vi "Find Parse State Queue from While Loop.vi"(8 "error in (no error)":errorcluster, 11 "WhileLoop in":refnum<vi>) -> (0 "error out":errorcluster, 1 "CaseStructure":refnum<vi>, 2 "Parse State Queue":refnum<vi>, 3 "WhileLoop out":refnum<vi>)   [LabVIEW 2020, in "CSM-Helper.lvclass"]
uses:
  CSM-Helper.lvclass
  CSM-Helper.lvclass/CSM-Helper.ctl
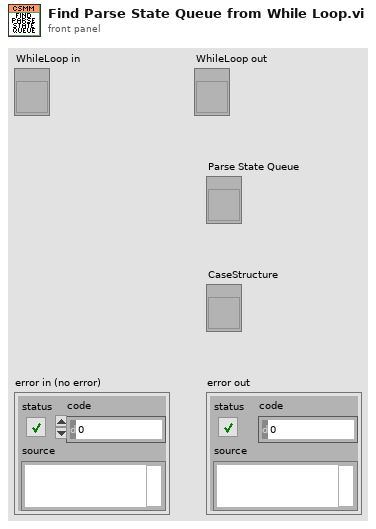
[diagram p1: front panel]
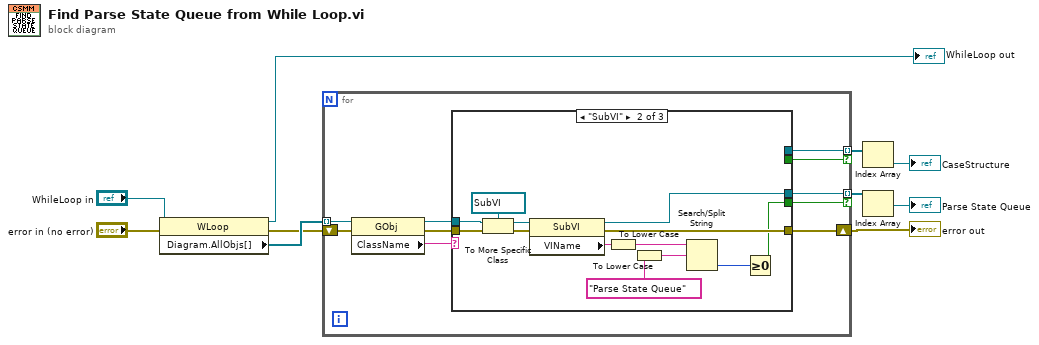
[diagram p0: block diagram]
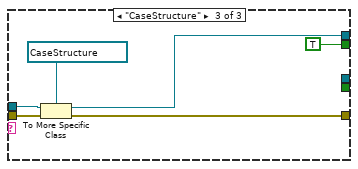
[diagram p3: hidden frame]
diagram:
  n1 = property on="Property Node" class="WLoop"(reference="WhileLoop in", error in="error in (no error)") -> (reference out=→"WhileLoop out":refnum<vi>, error out=w7:errorcluster, "Diagram.AllObjs[]"=w10:refnum<vi>[])
  n2 = for {
    tunnel: w10 -> [w20] mode=indexing
    shift-right: [w15] -> w6
    shift-left: w7 -> [w16]
    tunnel: [w14] -> w3 mode=indexing if=w11
    tunnel: [w13] -> w5 mode=indexing if=w12
    n3 = property class="GObj"(reference=w20, error in=w16) -> (reference out=w18:refnum<vi>, error out=w17:errorcluster, "ClassName"=w19:string)
    n4 = case shown="\"SubVI\"" w19 {
      tunnel: w18 -> [_ w33 w39]
      tunnel: w17 -> [w21 w32 w38]
      tunnel: [w21 w27 w37] -> w15
      tunnel: [_ w26 _] -> w14
      tunnel: [_ _ w36] -> w13
      tunnel: [_ _ TRUE] -> w12
      tunnel: [_ w22 _] -> w11
      frame Default {
      }
      frame "SubVI" {
        n5 = To More Specific Class(target class=refnum<vi> refnum ("SubVI Refnum"), reference=w33, error in=w32) -> (specific class reference=w31:refnum<vi>, error out=w30:errorcluster)
        n6 = property class="SubVI"(reference=w31, error in=w30) -> (reference out=w26:refnum<vi>, error out=w27:errorcluster, "VIName"=w29:string)
        n7 = To Lower Case(string=w29) -> (all lower case string=w24:string)
        n8 = To Lower Case(string="Parse State Queue" ("VI Name")) -> (all lower case string=w25:string)
        n9 = Search/Split String(string=w24, search string/char (-)=w25) -> (offset of match=w23:i32)  [unwired: 1 in, 2 out]
        n10 = Greater Or Equal To 0?(x=w23) -> (x >= 0?=w22:bool)
      }
      frame "CaseStructure" {
        n11 = To More Specific Class(target class=refnum<vi> refnum ("CaseSel Refnum"), reference=w39, error in=w38) -> (specific class reference=w36:refnum<vi>, error out=w37:errorcluster)
      }
    }
  }
  "error out" <- w6
  n12 = Index Array(array=w5) -> (element=→"CaseStructure":refnum<vi>)  [unwired: 1 in]
  n13 = Index Array(array=w3) -> (element=→"Parse State Queue":refnum<vi>)  [unwired: 1 in]
